vi "19-CompareAxes.vi"(0 "Match Translations z":i32[](array[numeric]), 4 "Match Translations y":i32[](array[numeric]), 6 "Match Translations x":i32[](array[numeric]), 7 "Rotation index":i32, 8 "Matches z":cluster{"Beacons":i32[][]}[](array[cluster]), 9 "Matches y":cluster{"Beacons":i32[][]}[](array[cluster]), 10 "Matches x":cluster{"Beacons":i32[][]}[](array[cluster])) -> (1 "max value":i32, 2 "Match Found?":bool, 3 "Match Info":T1)   [LabVIEW 2019, in "19.lvlib"]
uses:
  19.lvlib
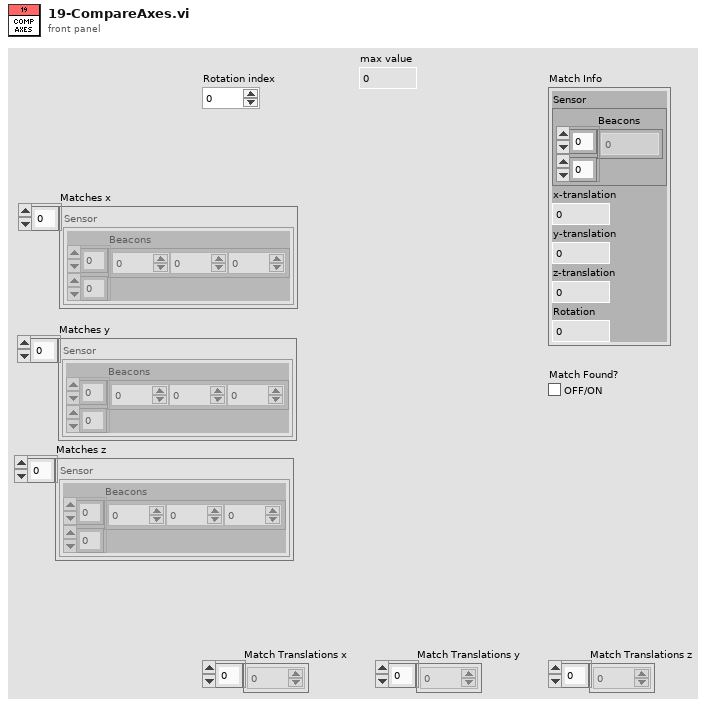
[diagram p1: front panel]
types:
  T1 = cluster{"Sensor":cluster{"Beacons":i32[][]}, "x-translation":i32, "y-translation":i32, "z-translation":i32, "Rotation":i32}
  T2 = cluster{cluster{"Beacons":i32[][]}, i32, i32, i32, "Rotation index":i32}
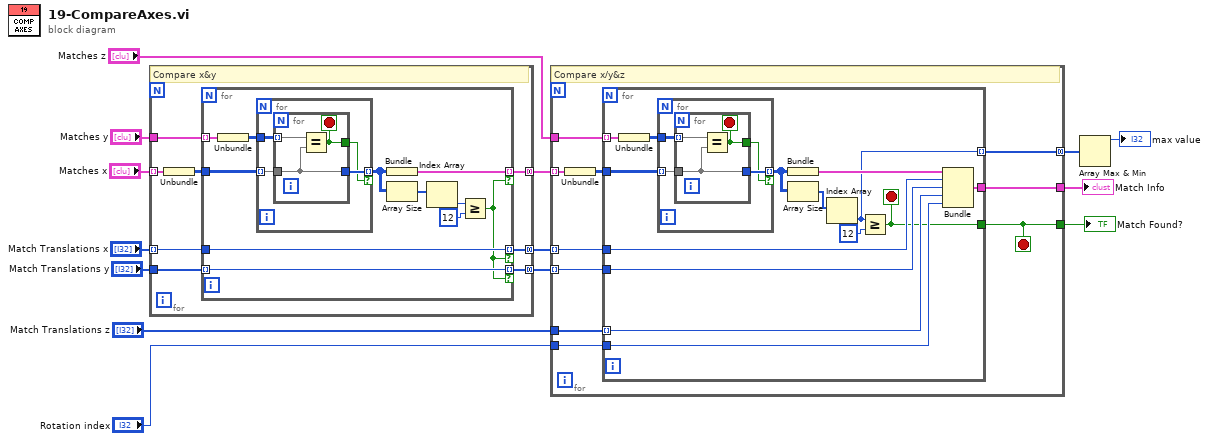
[diagram p0: block diagram]
diagram:
  n1 = for {
    tunnel: "Matches y" -> [w22]
    tunnel: "Match Translations y" -> [w18]
    tunnel: "Match Translations x" -> [w17] mode=indexing
    tunnel: [w16] -> w9 mode=concatenating
    tunnel: [w19] -> w6 mode=concatenating
    tunnel: "Matches x" -> [w21] mode=indexing
    tunnel: [w15] -> w8 mode=concatenating
    # "Compare x&y"
    n2 = Unbundle(w21) -> ("Beacons"=w20:i32[][])
    n3 = for {
      tunnel: w22 -> [w33] mode=indexing
      tunnel: w20 -> [w32]
      tunnel: [w26] -> w19 mode=indexing if=w23
      tunnel: [w25] -> w15 mode=indexing if=w23
      tunnel: w18 -> [w25] mode=indexing
      tunnel: w17 -> [w24]
      tunnel: [w24] -> w16 mode=indexing if=w23
      n4 = Unbundle(w33) -> ("Beacons"=w31:i32[][])
      n5 = for {
        tunnel: [w35] -> w27 mode=indexing if=w34
        tunnel: w32 -> [w37] mode=indexing
        tunnel: w31 -> [w36]
        n6 = for {
          tunnel: [w39] -> w35
          tunnel: w37 -> [w39]
          tunnel: w36 -> [w40] mode=indexing
          tunnel: [w38] -> w34
          stop <- w38 stop-if-true
          n7 = Equal?(x=w40, y=w39) -> (x = y?=w38:bool)
        }
      }
      n8 = Bundle("Beacons"=w27) -> (w26:cluster{"Beacons":i32[][]})  [unwired: 1 in]
      n9 = Array Size(array=w27) -> (size(s)=w30:i32[])
      n10 = Index Array(array=w30) -> (element=w29:i32)  [unwired: 1 in]
      n11 = Greater Or Equal?(x=w29, y=12) -> (x >= y?=w23:bool)
    }
  }
  n12 = for {
    tunnel: "Matches z" -> [w50]
    tunnel: "Match Translations z" -> [w46]
    tunnel: w9 -> [w45] mode=indexing
    tunnel: [w47] -> w4
    tunnel: w6 -> [w49] mode=indexing
    tunnel: w8 -> [w44] mode=indexing
    tunnel: "Rotation index" -> [w43]
    tunnel: [w42] -> w3
    tunnel: [w41] -> w2 mode=concatenating
    stop <- w42 stop-if-true
    # "Compare x/y&z"
    n13 = Unbundle(w49) -> ("Beacons"=w48:i32[][])
    n14 = for {
      tunnel: w50 -> [w64] mode=indexing
      tunnel: w48 -> [w63]
      tunnel: [w54] -> w47
      tunnel: w46 -> [w56] mode=indexing
      tunnel: w45 -> [w58]
      tunnel: w44 -> [w57]
      tunnel: w43 -> [w53]
      tunnel: [w52] -> w42
      tunnel: [w51] -> w41 mode=indexing
      stop <- w52 stop-if-true
      n15 = Unbundle(w64) -> ("Beacons"=w62:i32[][])
      n16 = for {
        tunnel: [w66] -> w59 mode=indexing if=w65
        tunnel: w63 -> [w68] mode=indexing
        tunnel: w62 -> [w67]
        n17 = for {
          tunnel: [w70] -> w66
          tunnel: w68 -> [w70]
          tunnel: w67 -> [w71] mode=indexing
          tunnel: [w69] -> w65
          stop <- w69 stop-if-true
          n18 = Equal?(x=w71, y=w70) -> (x = y?=w69:bool)
        }
      }
      n19 = Bundle("Beacons"=w59) -> (w55:cluster{"Beacons":i32[][]})  [unwired: 1 in]
      n20 = Array Size(array=w59) -> (size(s)=w61:i32[])
      n21 = Index Array(array=w61) -> (element=w51:i32)  [unwired: 1 in]
      n22 = Greater Or Equal?(x=w51, y=12) -> (x >= y?=w52:bool)
      n23 = Bundle(w55, w58, w57, w56, "Rotation index"=w53) -> (w54:T2)  [unwired: 1 in]
    }
  }
  "Match Info" <- w4
  "Match Found?" <- w3
  n24 = Array Max & Min(array=w2) -> (max value=→"max value":i32)  [unwired: 3 out]
